vi "Get Serial Number.vi"(8 "error in (no error)":errorcluster, 11 "Device in":refnum<class "Device.lvclass">) -> (0 "error out":errorcluster, 2 "Serial Number":string, 3 "Device out":refnum<class "Device.lvclass">)   [LabVIEW 2015]
uses:
  Device/Device.lvclass
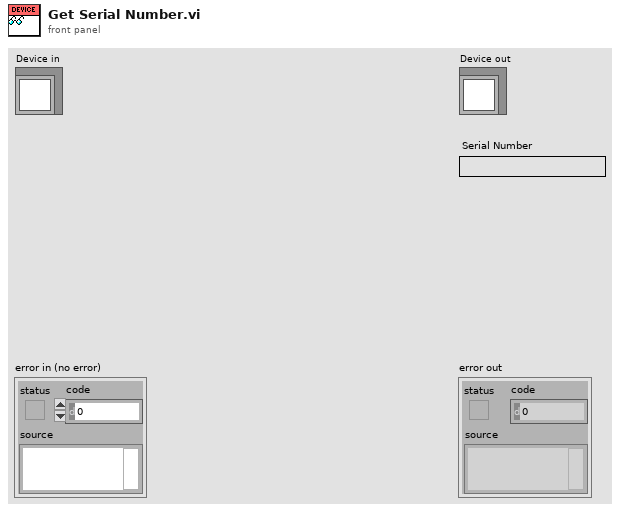
[diagram p1: front panel]
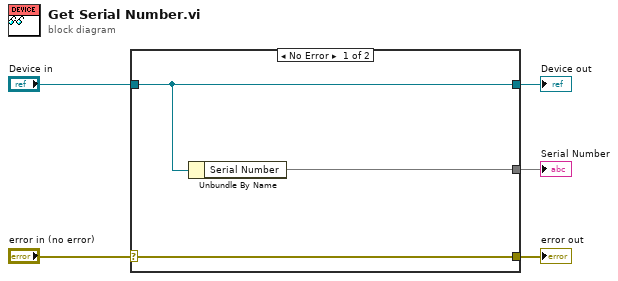
[diagram p0: block diagram]
diagram:
  n1 = case shown="No Error" "error in (no error)" {
    selector: "error in (no error)" -> [w8 w9]
    tunnel: [w8 w9] -> w4
    tunnel: [w7 w10] -> w2
    tunnel: "Device in" -> [w7 w10]
    tunnel: [w6 _] -> w1
    frame No Error {
      n2 = Unbundle By Name(w7) -> ("Serial Number"=w6)
    }
    frame Error {
    }
  }
  "error out" <- w4
  "Device out" <- w2
  "Serial Number" <- w1
